vi "Uninitialize.vi"(8 "error in (no error)":errorcluster) -> (0 "error out":errorcluster)   [LabVIEW 2025, in "Automotive Ethernet Bus Monitor UI.lvlib" / "lvwpcap.lvlib"]
doc: "This VI uninitializes the packet sniffer utility."
uses:
  lvwpcap.lvlib
  lvwpcap.dll
panel:
  # "Select Help»Show Context Help and move the cursor over the VI icon to display help for this VI."
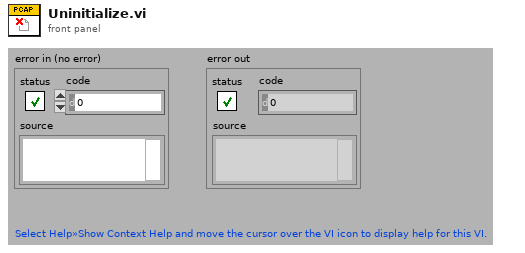
[diagram p1: front panel]
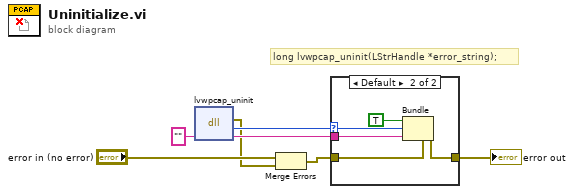
[diagram p0: block diagram]
diagram:
  # "long lvwpcap_uninit(LStrHandle *error_string);"
  n1 = dll-call lib="lvwpcap.*" fn="lvwpcap_uninit"("error_string"="") -> (error out=w2:errorcluster, "return type"=w7:i32, "error_string"=w6:string)  [unwired: 3 in, 1 out]
  n2 = Merge Errors("error in (no error)", w2) -> (w3:errorcluster)
  n3 = case shown="Default" w7 {
    selector: w7 -> [_ w12]
    tunnel: w6 -> [_ w11]
    tunnel: w3 -> [w8 w13]
    tunnel: [w8 w9] -> w4
    frame 0 {
    }
    frame Default {
      n4 = Bundle(cluster=w13, "status"=TRUE, "code"=w12, "source"=w11) -> (w9:errorcluster)
    }
  }
  "error out" <- w4
